vi "resetcolor.vi"(8 "error in (no error)":errorcluster, 9 "Color Box":u32(colorbox)=9868950, 11 "MulticolumnListbox in":refnum<vi>) -> (0 "error out":errorcluster, 3 "MulticolumnListbox out":refnum<vi>)   [LabVIEW 2022 SP3]
uses:
  <vilib>/Utility/miscctls.llb/LVRowAndColumnTypeDef.ctl
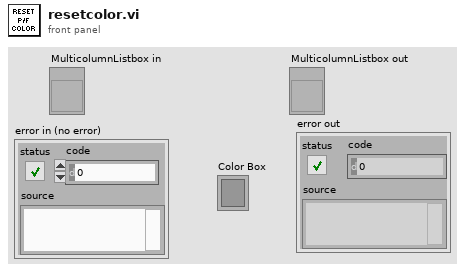
[diagram p1: front panel]
types:
  T1 = typedef "LVRowAndColumnTypeDef.ctl" = cluster{"Row":i32, "Column":i32}
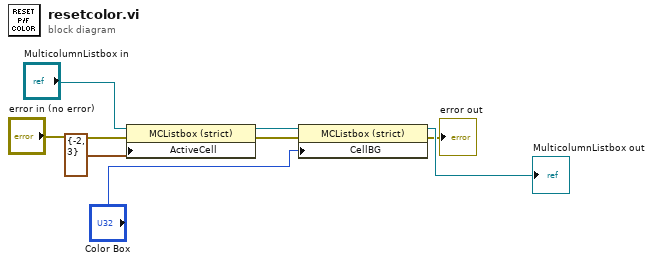
[diagram p0: block diagram]
diagram:
  n1 = property class="MCListbox (strict)"(reference="MulticolumnListbox in", error in="error in (no error)", "ActiveCell"=T1 {"Row"=-2, "Column"=3} ("Active Cell:Active Cell")) -> (reference out=w4:refnum<vi>, error out=w5:errorcluster)
  n2 = property class="MCListbox (strict)"(reference=w4, error in=w5, "CellBG"="Color Box") -> (reference out=→"MulticolumnListbox out":refnum<vi>, error out=→"error out":errorcluster)
